vi "SRV_ms Timer.vi"(2 "ms Previous Tick":u32, 3 "Pass Previous Error (T)":bool=TRUE, 4 "error in (no error)":errorcluster) -> (16 "ms Tick":u32, 17 "ms Diff":u32, 18 "error out":errorcluster)   [LabVIEW 2014]
doc: "(ms Diff) = (ms Tick) - (ms Previous Tick)\n\nUseful for timing sections of code and sub-VIs. Wire this VI in line with the error in and out both before and after the code to be timed.\n\n\nAuthor: Mike Schultz\n\n\nLogicPD, Inc\nwww.logicpd.com"
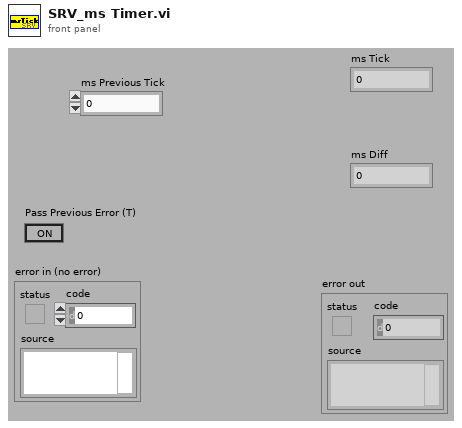
[diagram p1: front panel]
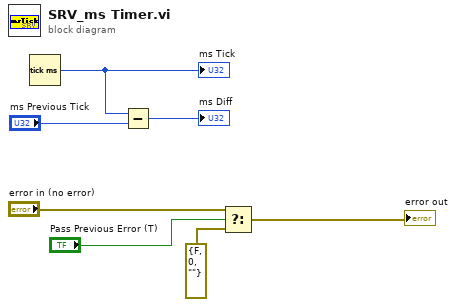
[diagram p0: block diagram]
diagram:
  n1 = Tick Count (ms)() -> (millisecond timer value=w7:u32)
  "ms Tick" <- w7
  n2 = Subtract(x=w7, y="ms Previous Tick") -> (x-y=→"ms Diff":u32)
  n3 = Select(t="error in (no error)", s="Pass Previous Error (T)", f=errorcluster {"status"=FALSE, "code"=0, "source"=""}) -> (s? t:f=→"error out":errorcluster)
